vi "ziGetCurrentParams.vi"(5 "PreampChannel (0)":dbl, 7 "ZCtrl (0)":dbl, 8 "Error In":errorcluster, 9 "Demodulator (0)":i32, 10 "Mode":T2(ring), 11 "Handle in":T1 {"Handle" format="0x%08x"; "Conn" format="0x%08x"}) -> (0 "Error Out":errorcluster, 1 "VGain":dbl, 2 "Gain R":dbl, 3 "Handle Out":T1 {"Handle" format="0x%08x"; "Conn" format="0x%08x"}, 4 "V (Vrms)":cdb, 6 "Imp50":bool)   [LabVIEW 2018, in "Zurich Instruments LabOne.lvlib"]
uses:
  Zurich Instruments LabOne.lvlib
  ziTypeHandle.ctl
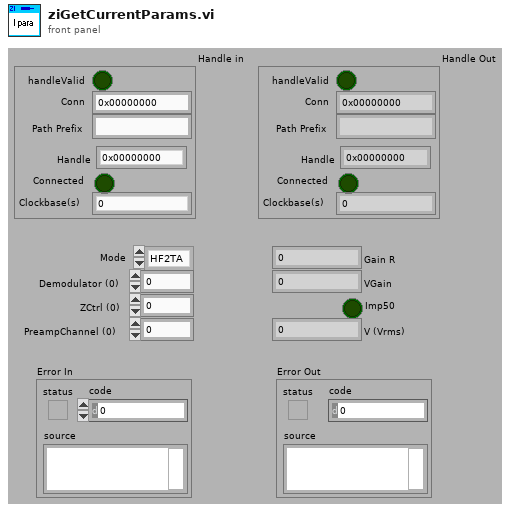
[diagram p1: front panel]
types:
  T1 = typedef "Zurich Instruments LabOne.lvlib/ziTypeHandle.ctl" = cluster{"handleValid":bool, "Conn":u64, "Path Prefix":string, "Handle":u64, "Connected":bool, "Clockbase(s)":dbl}
  T2 = enum16{"HF2TA", "HF2CA", "Int. Shunt", "Ext. Shunt"}
  T3 = typedef "Zurich Instruments LabOne.lvlib/ziTypeDemodSampleSingle.ctl" = cluster{"Timestamps (ticks)":u64, "X (Vrms)":dbl, "Y (Vrms)":dbl, "Osc Phase (deg)":dbl, "Freq (Hz)":dbl, "DIO":u32, "AuxIn0 (V)":dbl, "AuxIn1 (V)":dbl, "Trigger":u32}
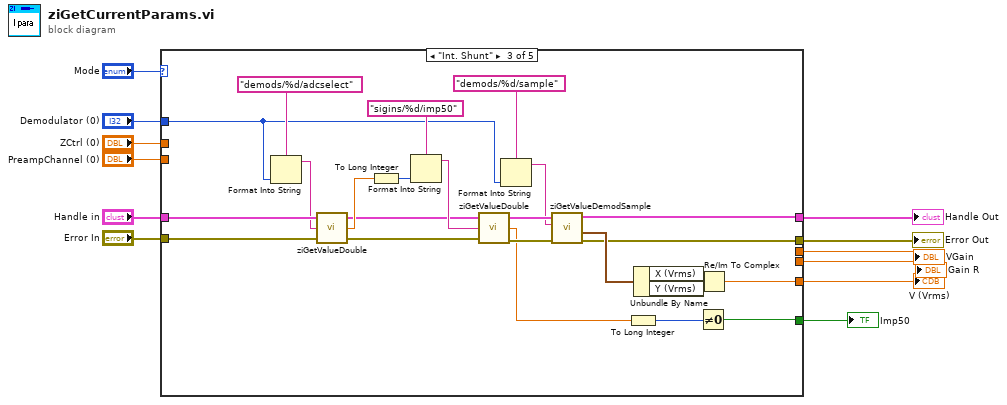
[diagram p0: block diagram]
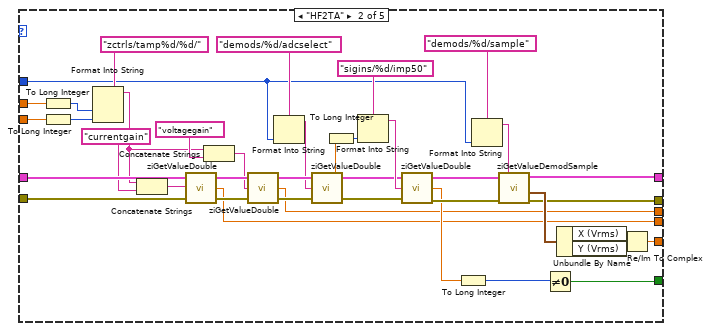
[diagram p3: hidden frame]
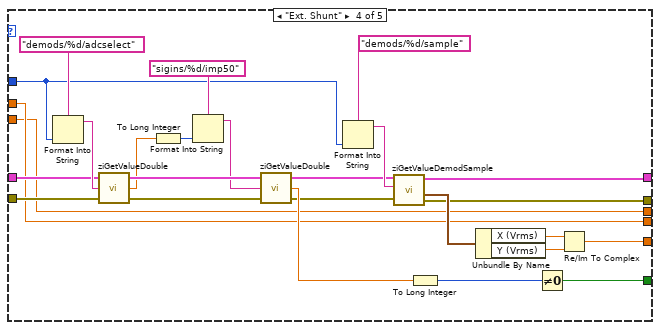
[diagram p4: hidden frame]
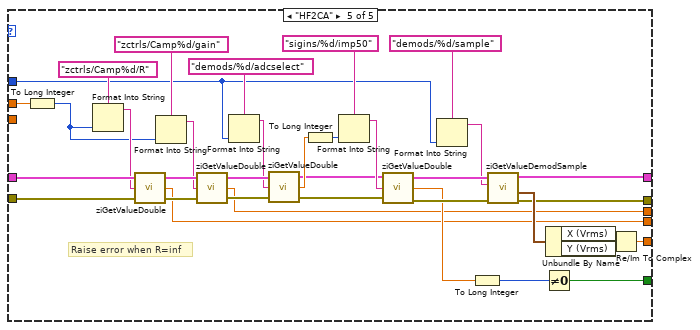
[diagram p5: hidden frame]
diagram:
  n1 = case shown="\"Int. Shunt\"" "Mode" {
    tunnel: "ZCtrl (0)" -> [_ w20 _ w82 w108]
    tunnel: "PreampChannel (0)" -> [_ w18 _ w81 _]
    tunnel: "Handle in" -> [w14 w54 w65 w87 w140]
    tunnel: [w14 w47 w74 w98 w129] -> w5
    tunnel: "Demodulator (0)" -> [_ w23 w59 w83 w113]
    tunnel: "Error In" -> [w13 w41 w64 w86 w123]
    tunnel: [w13 w40 w68 w97 w122] -> w12
    tunnel: [_ w30 w58 w101 w111] -> w9
    tunnel: [_ w29 _ w82 w110] -> w10
    tunnel: [_ w28 _ w81 w109] -> w11
    tunnel: [_ w15 w55 w79 w105] -> w1
    frame Default {
    }
    frame "HF2TA" {
      n2 = To Long Integer(number=w20) -> (32bit integer=w19:i32)
      n3 = To Long Integer(number=w18) -> (32bit integer=w17:i32)
      n4 = Format Into String(format string="zctrls/tamp%d/%d/", w19, w17) -> (resulting string=w22:string)  [unwired: 2 in, 1 out]
      n5 = Concatenate Strings(w22, "currentgain") -> (w21:string)
      n6 = call "ziGetValueDouble.vi"("error in"=w41, "Path"=w21, "Handle in"=w54) -> ("error out"=w52:errorcluster, "Value"=w29:dbl, "Handle out"=w53:T1)
      n7 = Concatenate Strings(w22, "voltagegain") -> (w24:string)
      n8 = call "ziGetValueDouble.vi"("error in"=w52, "Path"=w24, "Handle in"=w53) -> ("error out"=w37:errorcluster, "Value"=w28:dbl, "Handle out"=w38:T1)
      n9 = Format Into String(format string="demods/%d/adcselect", w23) -> (resulting string=w35:string)  [unwired: 2 in, 1 out]
      n10 = call "ziGetValueDouble.vi"("error in"=w37, "Path"=w35, "Handle in"=w38) -> ("error out"=w33:errorcluster, "Value"=w32:dbl, "Handle out"=w34:T1)
      n11 = To Long Integer(number=w32) -> (32bit integer=w31:i32)
      n12 = Format Into String(format string="sigins/%d/imp50", w31) -> (resulting string=w50:string)  [unwired: 2 in, 1 out]
      n13 = call "ziGetValueDouble.vi"("error in"=w33, "Path"=w50, "Handle in"=w34) -> ("error out"=w48:errorcluster, "Value"=w39:dbl, "Handle out"=w49:T1)
      n14 = To Long Integer(number=w39) -> (32bit integer=w16:i32)
      n15 = Format Into String(format string="demods/%d/sample", w23) -> (resulting string=w42:string)  [unwired: 2 in, 1 out]
      n16 = call "ziGetValueDemodSample.vi"("error in"=w48, "Path"=w42, "Handle In"=w49) -> ("error out"=w40:errorcluster, "Demod Sample Out"=w46:T3, "Handle Out"=w47:T1)  [unwired: 2 in]
      n17 = Not Equal To 0?(x=w16) -> (x != 0?=w15:bool)
      n18 = Unbundle By Name(w46) -> ("X (Vrms)"=w44:dbl, "Y (Vrms)"=w45:dbl)
      n19 = Re/Im To Complex(1:w45, 2:w44) -> (0:w30:cdb)
    }
    frame "Int. Shunt" {
      n20 = Format Into String(format string="demods/%d/adcselect", w59) -> (resulting string=w60:string)  [unwired: 2 in, 1 out]
      n21 = call "ziGetValueDouble.vi"("error in"=w64, "Path"=w60, "Handle in"=w65) -> ("error out"=w63:errorcluster, "Value"=w66:dbl, "Handle out"=w62:T1)
      n22 = To Long Integer(number=w66) -> (32bit integer=w61:i32)
      n23 = Format Into String(format string="sigins/%d/imp50", w61) -> (resulting string=w77:string)  [unwired: 2 in, 1 out]
      n24 = call "ziGetValueDouble.vi"("error in"=w63, "Path"=w77, "Handle in"=w62) -> ("error out"=w75:errorcluster, "Value"=w57:dbl, "Handle out"=w76:T1)
      n25 = Format Into String(format string="demods/%d/sample", w59) -> (resulting string=w69:string)  [unwired: 2 in, 1 out]
      n26 = call "ziGetValueDemodSample.vi"("error in"=w75, "Path"=w69, "Handle In"=w76) -> ("error out"=w68:errorcluster, "Demod Sample Out"=w73:T3, "Handle Out"=w74:T1)  [unwired: 2 in]
      n27 = To Long Integer(number=w57) -> (32bit integer=w56:i32)
      n28 = Unbundle By Name(w73) -> ("X (Vrms)"=w71:dbl, "Y (Vrms)"=w72:dbl)
      n29 = Not Equal To 0?(x=w56) -> (x != 0?=w55:bool)
      n30 = Re/Im To Complex(1:w72, 2:w71) -> (0:w58:cdb)
    }
    frame "Ext. Shunt" {
      n31 = Format Into String(format string="demods/%d/adcselect", w83) -> (resulting string=w95:string)  [unwired: 2 in, 1 out]
      n32 = call "ziGetValueDouble.vi"("error in"=w86, "Path"=w95, "Handle in"=w87) -> ("error out"=w92:errorcluster, "Value"=w91:dbl, "Handle out"=w93:T1)
      n33 = To Long Integer(number=w91) -> (32bit integer=w94:i32)
      n34 = Format Into String(format string="sigins/%d/imp50", w94) -> (resulting string=w89:string)  [unwired: 2 in, 1 out]
      n35 = call "ziGetValueDouble.vi"("error in"=w92, "Path"=w89, "Handle in"=w93) -> ("error out"=w84:errorcluster, "Value"=w96:dbl, "Handle out"=w85:T1)
      n36 = Format Into String(format string="demods/%d/sample", w83) -> (resulting string=w104:string)  [unwired: 2 in, 1 out]
      n37 = call "ziGetValueDemodSample.vi"("error in"=w84, "Path"=w104, "Handle In"=w85) -> ("error out"=w97:errorcluster, "Demod Sample Out"=w102:T3, "Handle Out"=w98:T1)  [unwired: 2 in]
      n38 = To Long Integer(number=w96) -> (32bit integer=w80:i32)
      n39 = Unbundle By Name(w102) -> ("X (Vrms)"=w100:dbl, "Y (Vrms)"=w99:dbl)
      n40 = Not Equal To 0?(x=w80) -> (x != 0?=w79:bool)
      n41 = Re/Im To Complex(1:w99, 2:w100) -> (0:w101:cdb)
    }
    frame "HF2CA" {
      # "Raise error when R=inf"
      n42 = To Long Integer(number=w108) -> (32bit integer=w107:i32)
      n43 = Format Into String(format string="zctrls/Camp%d/R", w107) -> (resulting string=w138:string)  [unwired: 2 in, 1 out]
      n44 = call "ziGetValueDouble.vi"("error in"=w123, "Path"=w138, "Handle in"=w140) -> ("error out"=w134:errorcluster, "Value"=w110:dbl, "Handle out"=w137:T1)
      n45 = Format Into String(format string="zctrls/Camp%d/gain", w107) -> (resulting string=w135:string)  [unwired: 2 in, 1 out]
      n46 = call "ziGetValueDouble.vi"("error in"=w134, "Path"=w135, "Handle in"=w137) -> ("error out"=w118:errorcluster, "Value"=w109:dbl, "Handle out"=w117:T1)
      n47 = Format Into String(format string="demods/%d/adcselect", w113) -> (resulting string=w116:string)  [unwired: 2 in, 1 out]
      n48 = call "ziGetValueDouble.vi"("error in"=w118, "Path"=w116, "Handle in"=w117) -> ("error out"=w114:errorcluster, "Value"=w119:dbl, "Handle out"=w115:T1)
      n49 = To Long Integer(number=w119) -> (32bit integer=w112:i32)
      n50 = Format Into String(format string="sigins/%d/imp50", w112) -> (resulting string=w132:string)  [unwired: 2 in, 1 out]
      n51 = call "ziGetValueDouble.vi"("error in"=w114, "Path"=w132, "Handle in"=w115) -> ("error out"=w130:errorcluster, "Value"=w121:dbl, "Handle out"=w131:T1)
      n52 = Format Into String(format string="demods/%d/sample", w113) -> (resulting string=w124:string)  [unwired: 2 in, 1 out]
      n53 = To Long Integer(number=w121) -> (32bit integer=w106:i32)
      n54 = call "ziGetValueDemodSample.vi"("error in"=w130, "Path"=w124, "Handle In"=w131) -> ("error out"=w122:errorcluster, "Demod Sample Out"=w128:T3, "Handle Out"=w129:T1)  [unwired: 2 in]
      n55 = Not Equal To 0?(x=w106) -> (x != 0?=w105:bool)
      n56 = Unbundle By Name(w128) -> ("X (Vrms)"=w126:dbl, "Y (Vrms)"=w127:dbl)
      n57 = Re/Im To Complex(1:w127, 2:w126) -> (0:w111:cdb)
    }
  }
  "Error Out" <- w12
  "VGain" <- w11
  "Gain R" <- w10
  "V (Vrms)" <- w9
  "Handle Out" <- w5
  "Imp50" <- w1
